vi "initialise.vi"(8 "error in (no error)":errorcluster, 11 "GenericPlugin in":refnum<class "ClockDL100201DAQmx.lvclass">) -> (0 "error out":errorcluster, 3 "GenericPlugin out":refnum<class "ClockDL100201DAQmx.lvclass">)   [LabVIEW 2010, in "ClockDL100201DAQmx.lvclass"]
doc: "The dynamic dispatch-version of this VI initalises the plug-in object by allocating and initalising any dynamic resources need."
uses:
  ClockDL100201DAQmx.lvclass
  GenericClock/GenericClock/GenericClock.lvclass
  ClockDL100201DAQmx.lvclass/ClockDL100201DAQmx.ctl
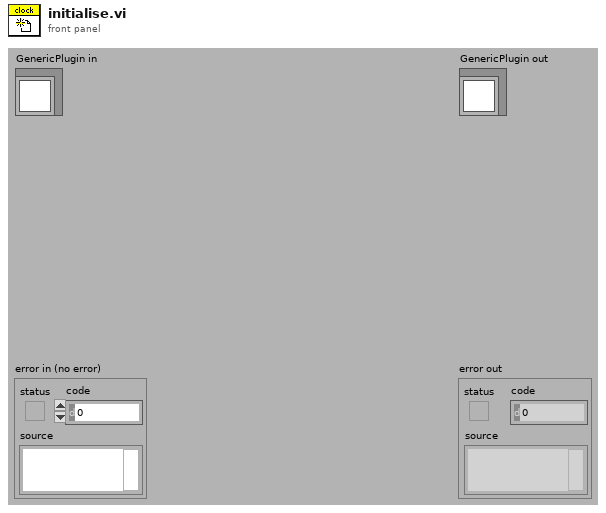
[diagram p1: front panel]
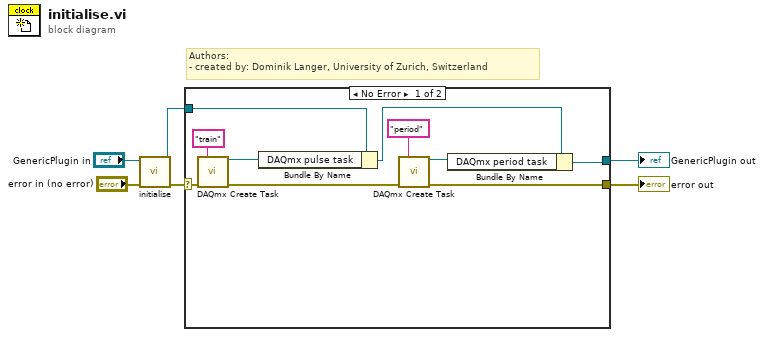
[diagram p0: block diagram]
diagram:
  # "Authors: \n- created by: Dominik Langer, University of Zurich, Switzerland"
  n1 = call-parent "initialise.vi"("error in (no error)"="error in (no error)", "GenericPlugin in"="GenericPlugin in") -> ("error out"=w4:errorcluster, "GenericPlugin out"=w3:refnum<class "ClockDL100201DAQmx.lvclass">)  [unwired: 8 in]
  n2 = case shown="No Error" w4 {
    selector: w4 -> [w16 w18]
    tunnel: w3 -> [w14 w17]
    tunnel: [w7 w18] -> w2
    tunnel: [w8 w17] -> w1
    frame No Error {
      n3 = call <vilib>:"DAQmx Create Task.vi"("new task name"="train", "error in"=w16) -> ("task out"=w15:refnum<k21>, "error out"=w11:errorcluster)  [unwired: 12 in]
      n4 = Bundle By Name(cluster=w14, "DAQmx pulse task"=w15) -> (w9:refnum<class "ClockDL100201DAQmx.lvclass">)
      n5 = call <vilib>:"DAQmx Create Task.vi"("new task name"="period", "error in"=w11) -> ("task out"=w10:refnum<k21>, "error out"=w7:errorcluster)  [unwired: 12 in]
      n6 = Bundle By Name(cluster=w9, "DAQmx period task"=w10) -> (w8:refnum<class "ClockDL100201DAQmx.lvclass">)
    }
    frame Error {
    }
  }
  "error out" <- w2
  "GenericPlugin out" <- w1
